vi "DuplicateSurface.vi"(8 "No Error":errorcluster, 11 "Surface [SDL_Surface *]":i64 format="%.0x") -> (0 "error out":errorcluster, 3 "Surface [SDL_Surface *]":i64 format="%.0x")   [LabVIEW 2024, in "SDL3.lvlib" / "Surface.lvlib"]
doc: "<B>Summary</B>\nCreates a new surface identical to the existing surface.\n\n<B>Remarks</B>\nIf the original surface has alternate images, the new surface will have a reference to them as well.\n\nThe returned surface should be freed with SDL_DestroySurface()."
uses:
  Surface.lvlib
  Lib/SDL3.dll
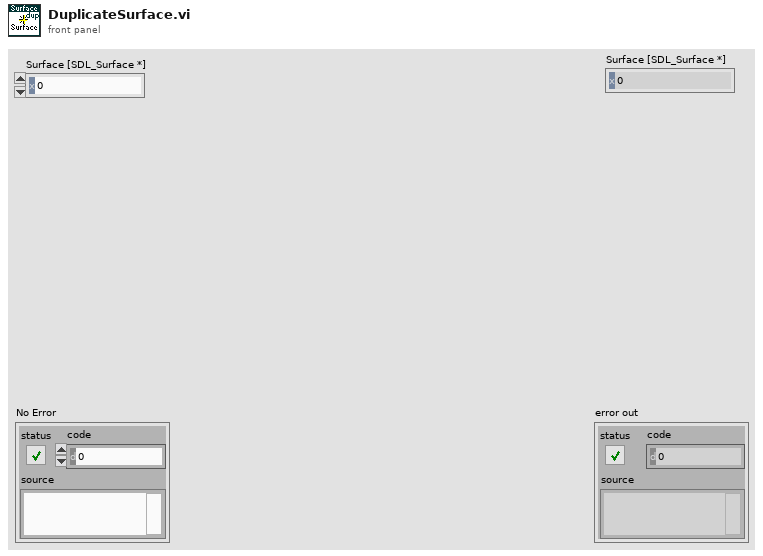
[diagram p1: front panel]
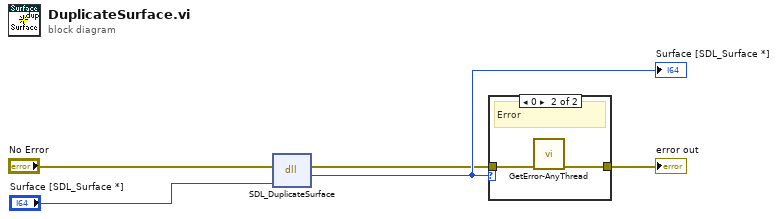
[diagram p0: block diagram]
diagram:
  n1 = dll-call lib="C:/Users/Thomas/Documents/Projects/LV-SDL3/Sources/SDL3/Lib/SDL3.*" fn="SDL_DuplicateSurface"(error in="No Error", "surface"="Surface [SDL_Surface *]") -> (error out=w1:errorcluster, "return type"=w3:i64)  [unwired: 3 in, 1 out]
  "Surface [SDL_Surface *]" <- w3
  n2 = case shown="0" w3 {
    tunnel: w1 -> [w6 w8]
    tunnel: [w6 w7] -> w4
    frame Default {
      # "Ok"
    }
    frame 0 {
      # "Error"
      n3 = call "GetError-AnyThread.vi"("No Error"=w8) -> ("Error Out"=w7:errorcluster)  [unwired: 10 in]
    }
  }
  "error out" <- w4
